vi "Calc Texture Stats v2.vi"(7 "Texture Dimensions":T1, 10 "UVs":cluster{"Top":T2, "Middle":T2, "Bottom":T2} {"Bottom"."v" min=0 max=1 step=0.1; "Bottom"."u" min=0 max=1 step=0.1; "Middle"."v" min=0 max=1 step=0.1; "Middle"."u" min=0 max=1 step=0.1; "Top"."v" min=0 max=1 step=0.1; "Top"."u" min=0 max=1 step=0.1}, 11 "Vertices":cluster{"Top":T1, "Middle":T1, "Bottom":T1}) -> ()   [LabVIEW 2022 SP3]
uses:
  Raster.lvlib
  UV.ctl
  Point 2D.ctl
panel:
  out "Start Deltas":T2 {"v" min=0 max=1 step=0.1; "u" min=0 max=1 step=0.1}
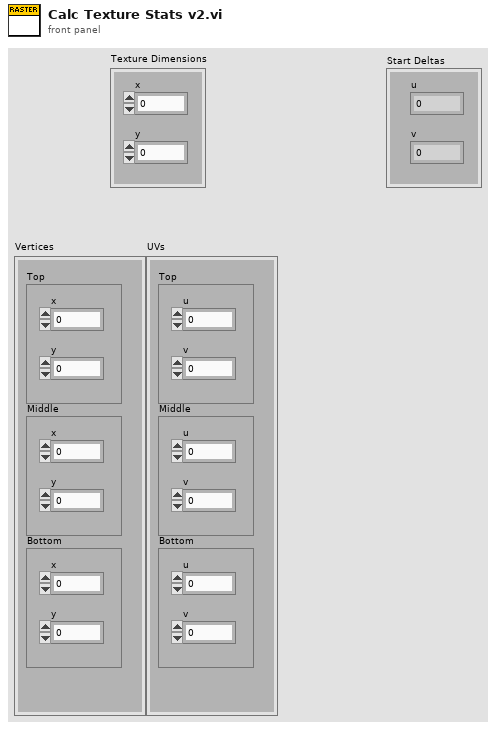
[diagram p1: front panel]
types:
  T1 = typedef "Raster.lvlib/Point 2D.ctl" = cluster{"x":i32, "y":i32}
  T2 = typedef "Raster.lvlib/UV.ctl" = cluster{"u":sgl, "v":sgl}
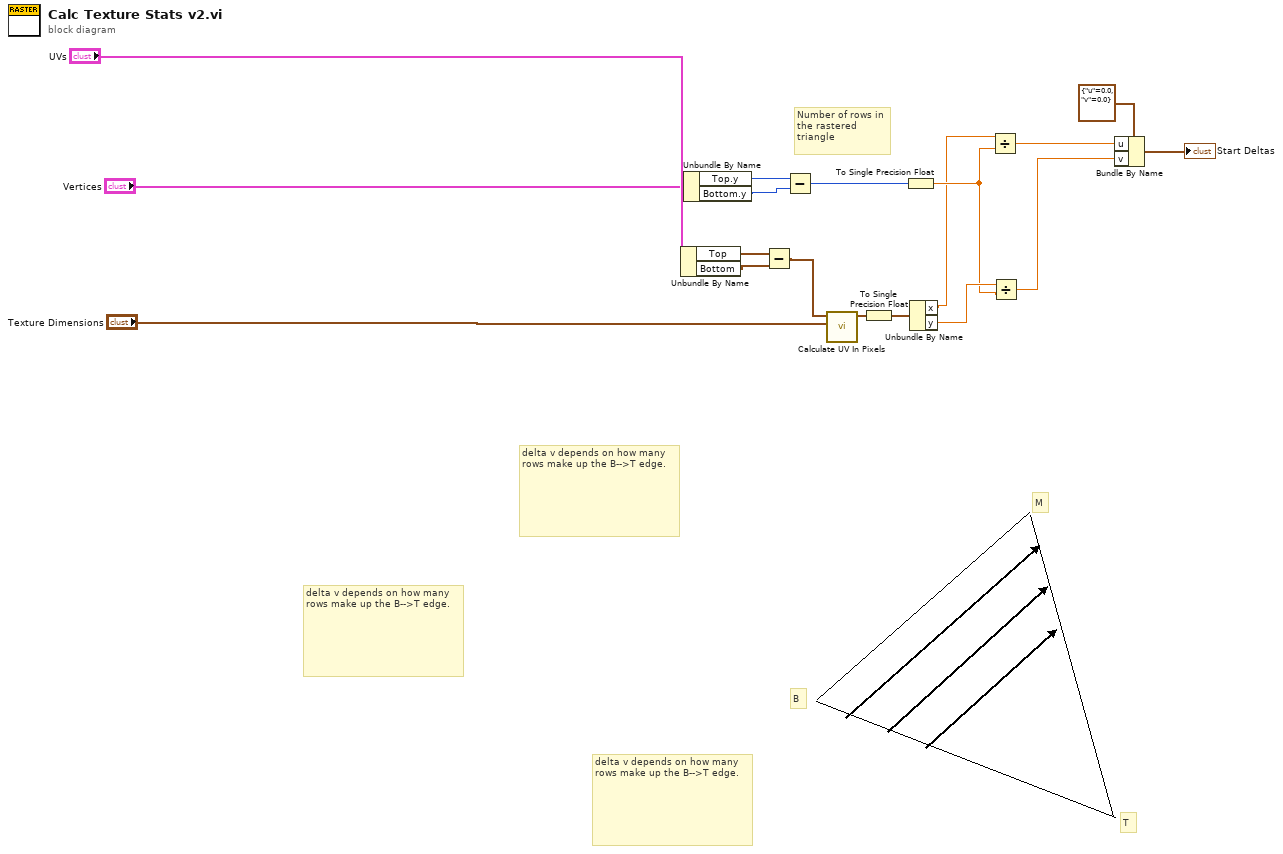
[diagram p0: block diagram]
diagram:
  # "delta v depends on how many rows make up the B-->T edge."
  # "Number of rows in the rastered triangle"
  # "delta v depends on how many rows make up the B-->T edge."
  # "T"
  # "M"
  # "B"
  # "delta v depends on how many rows make up the B-->T edge."
  n1 = Unbundle By Name("UVs") -> ("Top"=w11:T2, "Bottom"=w10:T2)
  n2 = Unbundle By Name("Vertices") -> ("Top.y"=w13:i32, "Bottom.y"=w12:i32)
  n3 = Subtract(x=w11, y=w10) -> (x-y=w9:T2)
  n4 = Subtract(x=w13, y=w12) -> (x-y=w8:i32)
  n5 = call "Calculate UV In Pixels.vi"(10:"Texture Dimensions", "UV"=w9) -> ("Pixels"=w6:T1)  [unwired: 9 in]
  n6 = To Single Precision Float(number=w6) -> (single precision float=w5:cluster{"x":sgl, "y":sgl})
  n7 = To Single Precision Float(number=w8) -> (single precision float=w3:sgl)
  n8 = Unbundle By Name(w5) -> ("x"=w2:sgl, "y"=w4:sgl)
  n9 = Divide(x=w2, y=w3) -> (x/y=w1:sgl)
  n10 = Divide(x=w4, y=w3) -> (x/y=w7:sgl)
  n11 = Bundle By Name(cluster=T2 {"u"=0.0, "v"=0.0} ("Start Deltas"), "u"=w1, "v"=w7) -> (→"Start Deltas":T2)
